vi "CryoServer Update Telemetry.vi"(8 "CryoServer Channels":map{string, T1}(c390), 9 "Values":dbl[](array[numeric]), 10 "Ch Names":string[](array[string]), 11 "Telem":T2) -> (3 "Telem out":T2)   [LabVIEW 2021]
uses:
  CryoServer Telemetry Map.ctl
  CryoServer Channel Mapping.ctl
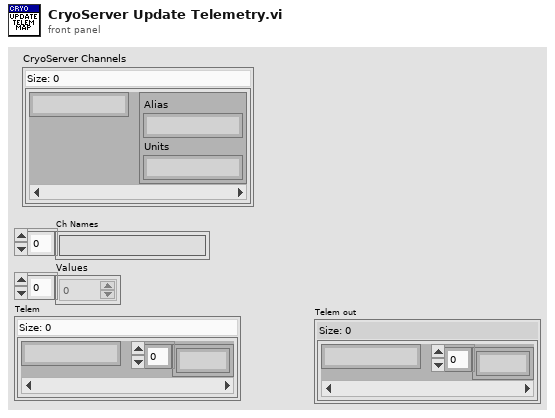
[diagram p1: front panel]
types:
  T1 = typedef "CryoServer Channel Mapping.ctl" = cluster{"Alias":string, "Units":string}
  T2 = typedef "CryoServer Telemetry Map.ctl" = map{string, dbl[]}
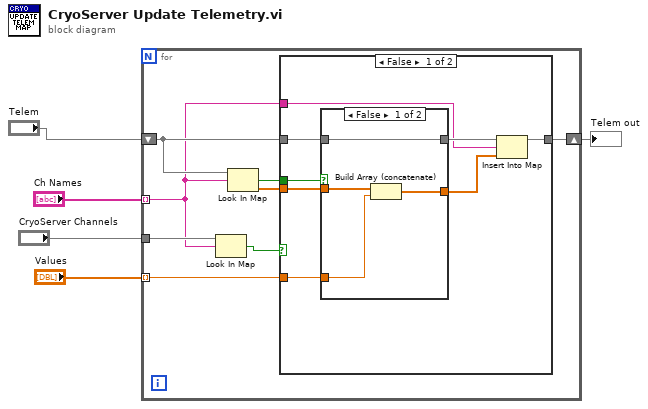
[diagram p0: block diagram]
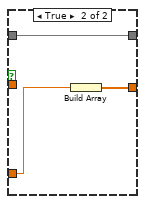
[diagram p2: hidden frame]
diagram:
  n1 = for {
    shift-right: [w9] -> w2
    shift-left: "Telem" -> [w10]
    tunnel: "Ch Names" -> [w7] mode=indexing
    tunnel: "Values" -> [w11] mode=indexing
    tunnel: "CryoServer Channels" -> [w8]
    n2 = Look In Map(map=w8, key=w7) -> (key not found?=w6:bool)  [unwired: 1 in, 1 out]
    n3 = Look In Map(map=w10, key=w7) -> (key not found?=w13:bool, value=w12:dbl[])  [unwired: 1 in]
    n4 = case shown="False" w6 {
      tunnel: w13 -> [w21 _]
      tunnel: w12 -> [w20 _]
      tunnel: w11 -> [w19 _]
      tunnel: w10 -> [w18 w29]
      tunnel: [w15 w29] -> w9
      tunnel: w7 -> [w14 _]
      frame False {
        n5 = case shown="False" w21 {
          tunnel: w20 -> [w25 _]
          tunnel: w19 -> [w24 w26]
          tunnel: w18 -> [w23 w28]
          tunnel: [w23 w28] -> w17
          tunnel: [w22 w27] -> w16
          frame False {
            n6 = Build Array (concatenate)(w25, w24) -> (w22:dbl[])
          }
          frame True {
            n7 = Build Array(w26) -> (w27:dbl[])
          }
        }
        n8 = Insert Into Map(map in=w17, key=w14, value=w16) -> (map out=w15:T2)  [unwired: 2 out]
      }
      frame True {
      }
    }
  }
  "Telem out" <- w2
